vi "lightControl_v2.vi"(1 "Boolean":bool, 2 "Baud Rate":dbl=57600.0, 3 "Channel":u8=2, 4 "VISA resource name":refnum<visa-resource-name>="COM4") -> (0 "Boolean 2":bool)   [LabVIEW 2015]
panel:
  in  "Stop":bool
  in  "Intensity (0-100%)":dbl=100.0
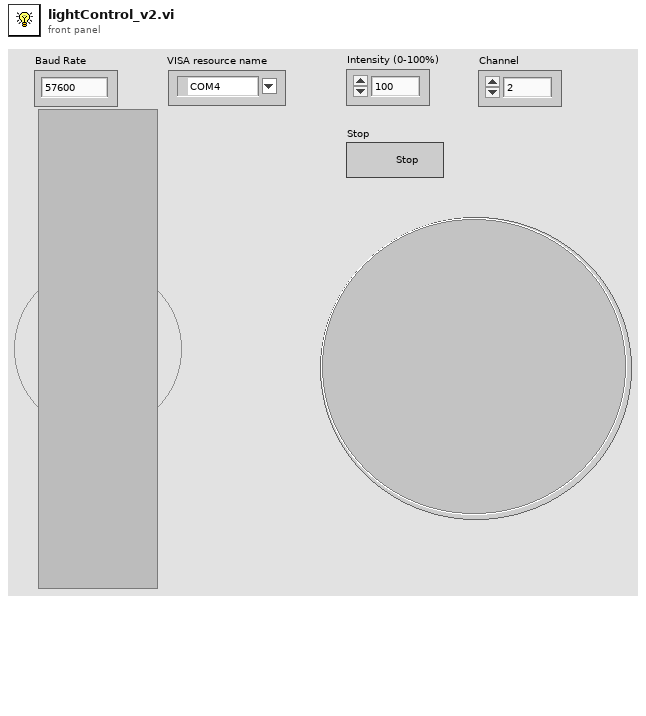
[diagram p1: front panel]
types:
  T1 = enum16{"Wait Off", "Wait On", "Turn Off", "Turn On"}
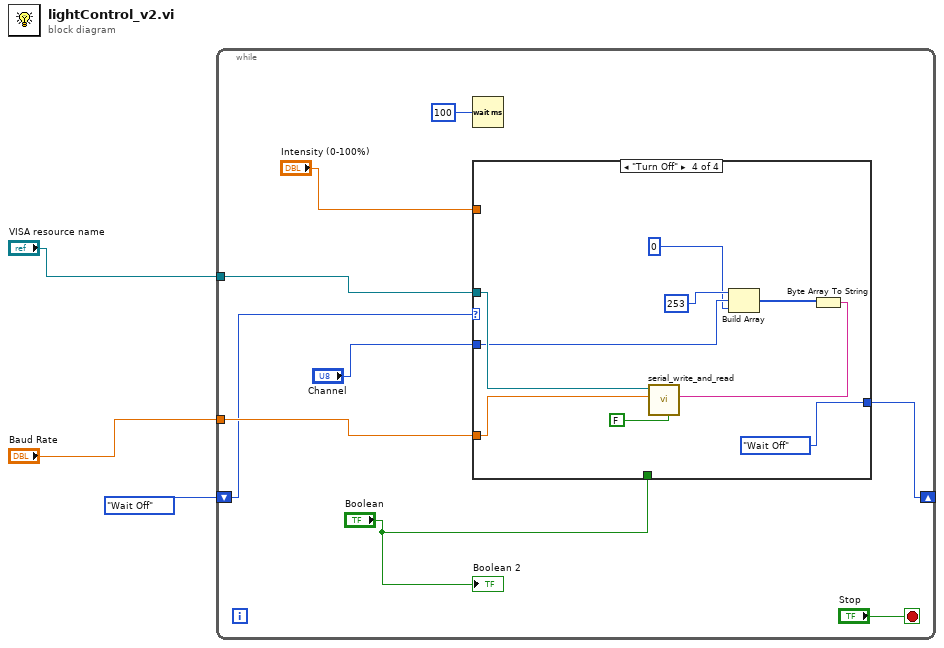
[diagram p0: block diagram]
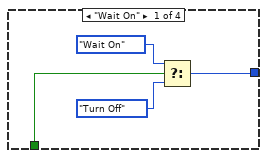
[diagram p2: hidden frame]
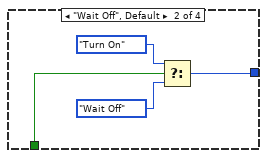
[diagram p3: hidden frame]
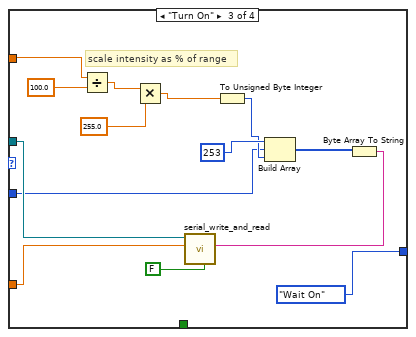
[diagram p4: hidden frame]
diagram:
  n1 = while {
    tunnel: "VISA resource name" -> [w12]
    tunnel: "Baud Rate" -> [w11]
    shift-right: [w8] -> _
    shift-left: T1."Wait Off" -> [w10]
    stop <- "Stop" stop-if-true
    n2 = Wait (ms)(milliseconds to wait=u32 100) -> ()  [unwired: 1 out]
    n3 = case shown="\"Turn Off\"" w10 {
      tunnel: w12 -> [_ _ w23 w38]
      tunnel: w11 -> [_ _ w24 w39]
      tunnel: "Intensity (0-100%)" -> [_ _ w30 _]
      tunnel: "Boolean" -> [w14 w20 _ _]
      tunnel: [w13 w17 T1."Wait On" T1."Wait Off"] -> w8
      tunnel: "Channel" -> [_ _ w21 w36]
      frame "Wait On" {
        n4 = Select(t=T1."Wait On", s=w14, f=T1."Turn Off") -> (s? t:f=w13:T1)
      }
      frame "Wait Off", Default {
        n5 = Select(t=T1."Turn On", s=w20, f=T1."Wait Off") -> (s? t:f=w17:T1)
      }
      frame "Turn On" {
        # "scale intensity as % of range"
        n6 = Divide(x=w30, y=100.0) -> (x/y=w32:dbl)
        n7 = Multiply(x=w32, y=255.0) -> (x*y=w34:dbl)
        n8 = To Unsigned Byte Integer(number=w34) -> (unsigned 8bit integer=w27:u8)
        n9 = Build Array(u8 253 ("element"), w21, w27) -> (w29:u8[])
        n10 = Byte Array To String(unsigned byte array=w29) -> (string=w25:string)
        n11 = call "serial_write_and_read.vi"("VISA resource name"=w23, "baud rate"=w24, "read"=FALSE, "string to write"=w25) -> ()  [unwired: 6 in, 1 out]
      }
      frame "Turn Off" {
        n12 = Build Array(u8 253 ("element"), w36, u8 0 ("element")) -> (w43:u8[])
        n13 = Byte Array To String(unsigned byte array=w43) -> (string=w40:string)
        n14 = call "serial_write_and_read.vi"("VISA resource name"=w38, "baud rate"=w39, "read"=FALSE, "string to write"=w40) -> ()  [unwired: 6 in, 1 out]
      }
    }
    "Boolean 2" <- "Boolean"
  }
